vi "SPOL_temps2.vi"() -> ()   [LabVIEW 2009]
uses:
  <vilib>/Utility/file.llb/Write To Spreadsheet File (string).vi
panel:
  in  "Data Direcory":string="/home/operator/data/spol_temps/"
  out "Data File":path
  out "Temperatures":T1(graph)
  out "Next Sample":dbl format="%.3g"
  in  "loop time(ms)":u32=250
  out "Samples":i32
  in  "stop":bool
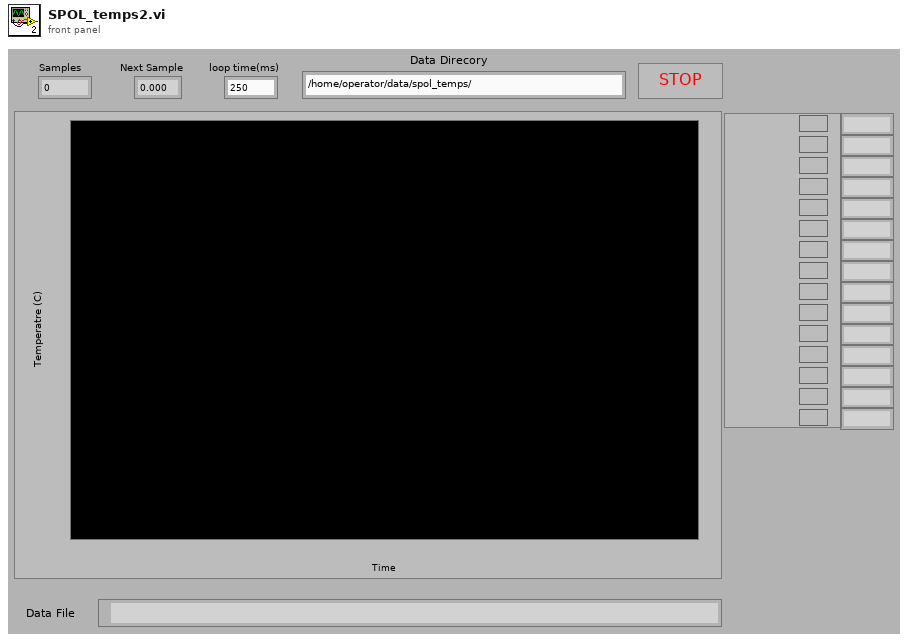
[diagram p1: front panel]
types:
  T1 = cluster{"[0]":dbl, "[1]":dbl, "[2]":dbl, "[3]":dbl, "[4]":dbl, "[5]":dbl, "[6]":dbl, "[7]":dbl, "[8]":dbl, "[9]":dbl, "[10]":dbl, "[11]":dbl, "[12]":dbl, "[13]":dbl, "[14]":dbl}
  T2 = cluster{"[0]":dbl, "[1]":dbl, "[2]":dbl, "[3]":dbl, "[4]":dbl, "[5]":dbl, "[6]":dbl, "[7]":dbl, "[8]":dbl, "[9]":dbl, "[10]":dbl, "[11]":dbl, "[12]":dbl, "[13]":dbl, "[14]":dbl}[]
  T3 = cluster{"Temperatures[0]":dbl, "Temperatures[1]":dbl, "Temperatures[2]":dbl, "Temperatures[3]":dbl, "Temperatures[4]":dbl, "Temperatures[5]":dbl, "Temperatures[6]":dbl, "Temperatures[7]":dbl, "Temperatures[8]":dbl, "Temperatures[9]":dbl, "Temperatures[10]":dbl, "Temperatures[11]":dbl, "Temperatures[12]":dbl, "Temperatures[13]":dbl, "Temperatures[14]":dbl}
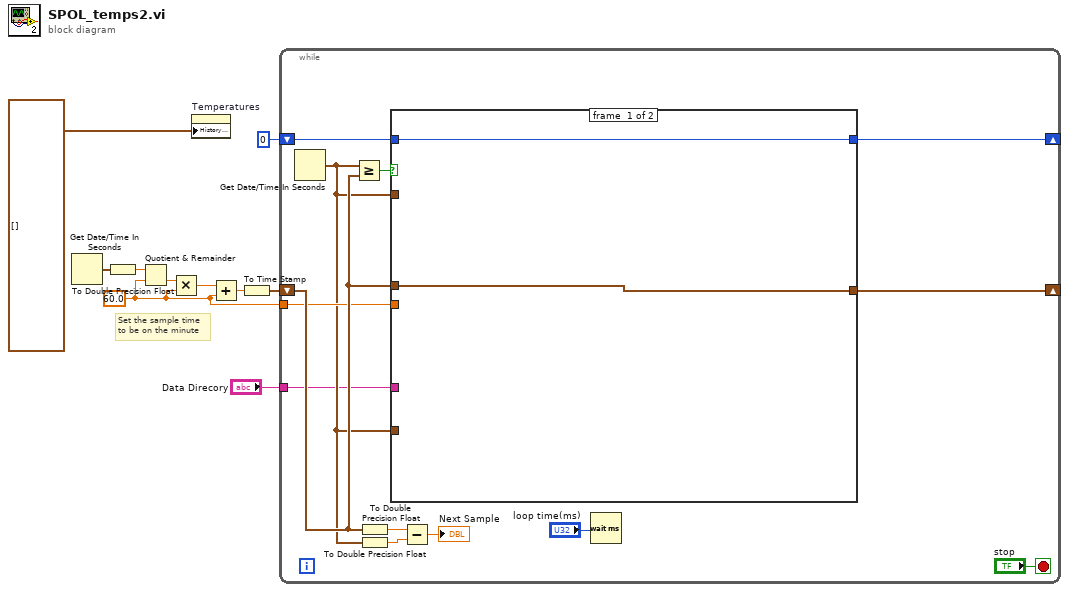
[diagram p0: block diagram]
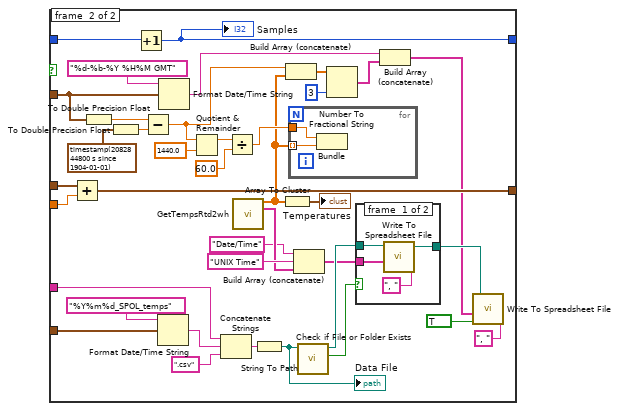
[diagram p2: hidden frame]
diagram:
  w2 = 60.0 ("y")
  # "Set the sample time\nto be on the minute"
  n1 = Get Date/Time In Seconds() -> (seconds since 1Jan1904=w4:timestamp)
  n2 = To Double Precision Float(number=w4) -> (double precision float=w10:dbl)
  n3 = Quotient & Remainder(x=w10, y=w2) -> (floor(x/y)=w8:dbl)  [unwired: 1 out]
  n4 = Multiply(x=w8, y=w2) -> (x*y=w9:dbl)
  n5 = property on="Temperatures" class="WFChart (strict)"("History Data"=T2 []) -> ()  [unwired: 2 in, 2 out]
  n6 = Add(x=w9, y=w2) -> (x+y=w7:dbl)
  n7 = To Time Stamp(1:w7) -> (0:w5:timestamp)
  n8 = while {
    tunnel: w2 -> [w18]
    shift-right: [w23] -> _
    shift-left: w5 -> [w19]
    shift-right: [w21] -> _
    shift-left: 0 -> [w22]
    tunnel: "Data Direcory" -> [w11]
    stop <- "stop" stop-if-true
    n9 = Get Date/Time In Seconds() -> (seconds since 1Jan1904=w16:timestamp)
    n10 = Greater Or Equal?(x=w16, y=w19) -> (x >= y?=w20:bool)
    n11 = To Double Precision Float(number=w19) -> (double precision float=w15:dbl)
    n12 = To Double Precision Float(number=w16) -> (double precision float=w14:dbl)
    n13 = case shown="True" w20 {
      tunnel: w19 -> [w25 w60]
      tunnel: [w25 w63] -> w23
      tunnel: w22 -> [w24 w62]
      tunnel: [w24 w61] -> w21
      tunnel: w16 -> [_ w39]
      tunnel: w18 -> [_ w59]
      tunnel: w16 -> [_ w45]
      tunnel: w11 -> [_ w26]
      frame #0 {
      }
      frame #1 {
        n14 = Add(x=w60, y=w59) -> (x+y=w63:timestamp)
        n15 = To Double Precision Float(number=w39) -> (double precision float=w40:dbl)
        n16 = To Double Precision Float(number=timestamp(2082844800 s since 1904-01-01)) -> (double precision float=w41:dbl)
        n17 = Increment(x=w62) -> (x+1=w61:i32)
        "Samples" <- w61
        n18 = Subtract(x=w40, y=w41) -> (x-y=w29:dbl)
        n19 = Format Date/Time String(time format string (%c)="%Y%m%d_SPOL_temps", seconds (now)=w45) -> (date/time string=w49:string)  [unwired: 1 in]
        n20 = Format Date/Time String(time format string (%c)="%d-%b-%Y %H%M GMT", seconds (now)=w39) -> (date/time string=w36:string)  [unwired: 1 in]
        n21 = Quotient & Remainder(x=w29, y=1440.0) -> (x-y*floor(x/y)=w31:dbl)  [unwired: 1 out]
        n22 = Concatenate Strings(w26, w49, ".csv" ("string")) -> (w51:string)
        n23 = Divide(x=w31, y=60.0) -> (x/y=w28:dbl)
        n24 = call "GetTempsRtd2wh.vi"() -> ("Temperatures"=w27:dbl[], "Variables"=w53:string[])  [unwired: 12 in, 2 out]
        n25 = String To Path(string=w51) -> (path=w46:path)
        "Data File" <- w46
        n26 = Array To Cluster(array=w27) -> (cluster=→"Temperatures":T3)
        n27 = Build Array (concatenate)(w29, w27) -> (w38:dbl[])
        n28 = for {
          tunnel: w28 -> [w65]
          tunnel: w27 -> [w64] mode=indexing
          n29 = Bundle(w65, "Value"=w64) -> ()  [unwired: 1 in, 1 out]
        }
        n30 = Build Array (concatenate)("Date/Time" ("element"), "UNIX Time", w53) -> (w52:string[])
        n31 = call <vilib>:"Check if File or Folder Exists.vi"("path"=w46) -> ("file or folder exists?"=w56:bool, "dup path"=w57:path)  [unwired: 8 in, 1 out]
        n32 = Number To Fractional String(number=w38, precision (6)=i16 3) -> (F-format string=w37:string[])  [unwired: 2 in]
        n33 = case shown="True" w56 {
          tunnel: w57 -> [w69 w70]
          tunnel: w52 -> [w68 _]
          tunnel: [w67 w70] -> w55
          frame #0 {
            n34 = call-poly <vilib>:"Write To Spreadsheet File.vi"("delimiter (\\t)"=", " ("delimiter (\\t)"), "1D data"=w68, "file path (dialog if empty)"=w69) -> ("new file path (Not A Path if cancelled)"=w67:path)  [unwired: 5 in]
          }
          frame #1 {
          }
        }
        n35 = Build Array (concatenate)(w36, w37) -> (w35:string[])
        n36 = call-poly <vilib>:"Write To Spreadsheet File.vi"("delimiter (\\t)"=", " ("delimiter (\\t)"), "append to file? (new file:F)"=TRUE, "1D data"=w35, "file path (dialog if empty)"=w55) -> ()  [unwired: 4 in, 1 out]
      }
    }
    n37 = Subtract(x=w15, y=w14) -> (x-y=→"Next Sample":dbl)
    n38 = Wait (ms)(milliseconds to wait="loop time(ms)") -> ()  [unwired: 1 out]
  }
